vi "Is Error.vi"(11 "Base Event jettl in":refnum<class "Base Event jettl.lvclass">) -> (3 "Base Event jettl out":refnum<class "Base Event jettl.lvclass">)   [LabVIEW 2021, in "jettl.lvlib" / "Base Event jettl.lvlib" / "Base Event jettl.lvclass"]
uses:
  Base Event jettl.lvclass
  State/Error State/Error State.lvclass
  C:/git/jettl/src/jettl/Base Event jettl/State/State/State.lvclass
  Base Event jettl.lvclass/Base Event jettl.ctl
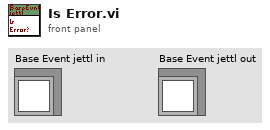
[diagram p1: front panel]
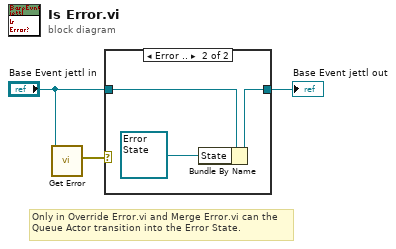
[diagram p0: block diagram]
diagram:
  # "Only in Override Error.vi and Merge Error.vi can the Queue Actor transition into the Error State."
  n1 = call-dynamic "Get Error.vi"("Base Event jettl in"="Base Event jettl in") -> ("Error"=w1:errorcluster)  [unwired: 10 in]
  n2 = case shown="Error .." w1 {
    tunnel: [w4 w6] -> w3
    tunnel: "Base Event jettl in" -> [w4 w7]
    frame No Error {
    }
    frame Error {
      n3 = Bundle By Name(cluster=w7, "State"=refnum<class "Error State.lvclass"> refnum ("jettl.lvlib:Error Event State.lvclass")) -> (w6:refnum<class "Base Event jettl.lvclass">)
    }
  }
  "Base Event jettl out" <- w3
